vi "Create.vi"(8 "error in (no error)":errorcluster, 11 "U32 array in":u32[](array[numeric])) -> (0 "error out":errorcluster, 3 "Uint32Array out":refnum<class "Uint32Array.lvclass">)   [LabVIEW 2012, in "MDSplus.lvlib" / "Uint32Array.lvclass"]
uses:
  <vilib>/MDSplus/Classes/Data_Class/Array_Class/Uint32Array_Class/Uint32Array.lvclass
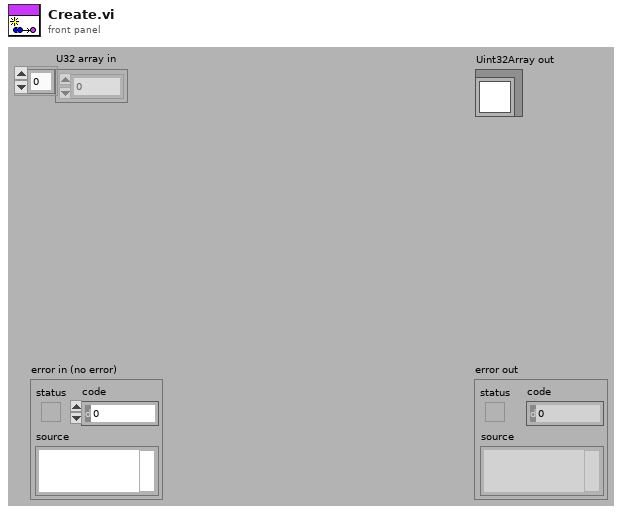
[diagram p1: front panel]
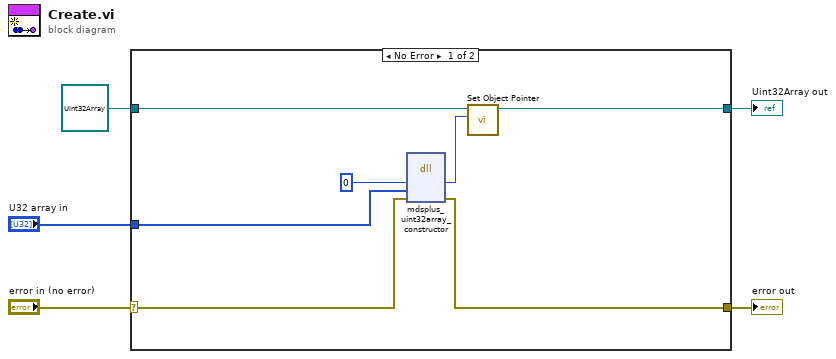
[diagram p0: block diagram]
diagram:
  n1 = case shown="No Error" "error in (no error)" {
    selector: "error in (no error)" -> [w10 w14]
    tunnel: [w6 w14] -> w4
    tunnel: [w8 w13] -> w2
    tunnel: refnum<class "Uint32Array.lvclass"> refnum ("Float32 in") -> [w9 w13]
    tunnel: "U32 array in" -> [w7 _]
    frame No Error {
      n2 = dll-call lib="MDSobjectsLVShr" fn="mdsplus_uint32array_constructor"("lvUint32ArrayPtrOut"=i64 0 ("lvTreePtr"), "lvUIntArrHdlIn"=w7, "error"=w10) -> ("lvUint32ArrayPtrOut"=w11:i64, "error"=w6:errorcluster)  [unwired: 5 in, 2 out]
      n3 = call-dynamic "Set Object Pointer.vi"("Object Pointer"=w11, "Data in"=w9) -> ("Data out"=w8:refnum<class "Uint32Array.lvclass">)  [unwired: 9 in]
    }
    frame Error {
    }
  }
  "error out" <- w4
  "Uint32Array out" <- w2
